vi "Drive Train Global.vi"() -> ()   [LabVIEW 2014]
panel:
  in  "Drive Train":T1
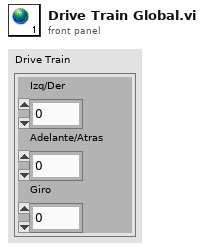
[diagram p1: front panel]
types:
  T1 = cluster{"Izq/Der":dbl, "Adelante/Atras":dbl, "Giro":dbl}
diagram:
